vi "GoTo.vi"(7 "theta":dbl, 8 "error in (no error)":errorcluster, 9 "Position":cluster{"X":dbl, "Y":dbl, "Theta":dbl}, 10 "y path":i32[](array[numeric]), 11 "x path":i32[](array[numeric])) -> (0 "Error/Flow Out":errorcluster, 1 "New Position":cluster{"X":dbl, "Y":dbl, "Theta":dbl})   [LabVIEW 2018]
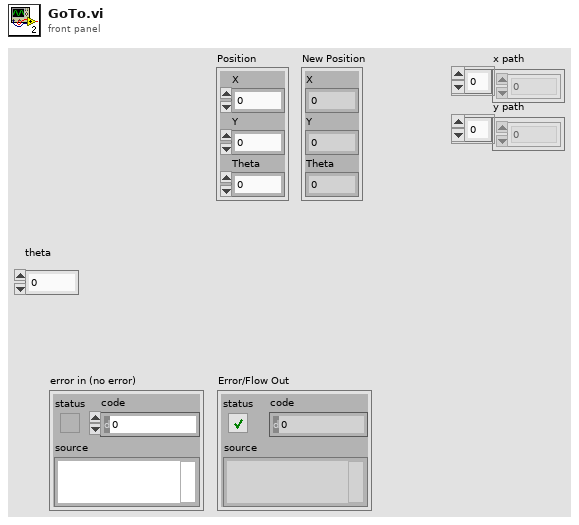
[diagram p1: front panel]
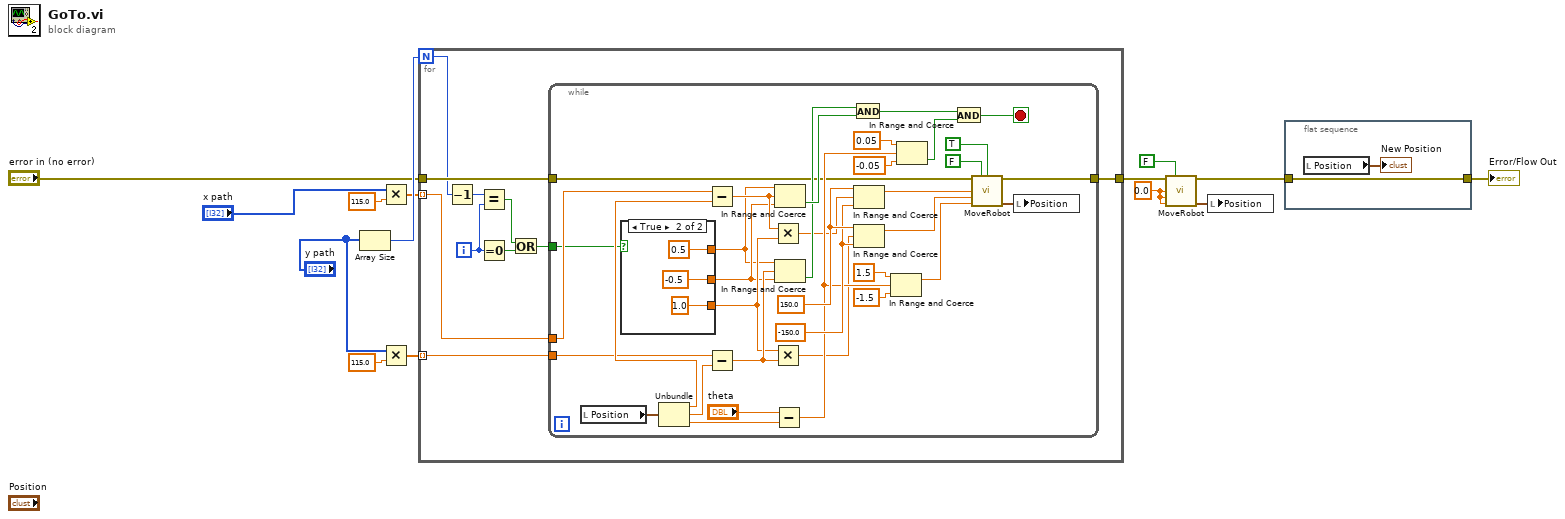
[diagram p0: block diagram]
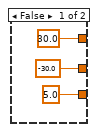
[diagram p2: hidden frame]
diagram:
  w6 = 0.0 ("x (mm/s)")
  n1 = Array Size(array="y path") -> (size(s)=w10:i32)
  n2 = Multiply(x="x path", y=115.0) -> (x*y=w8:dbl[])
  n3 = Multiply(x="y path", y=115.0) -> (x*y=w9:dbl[])
  n4 = for {
    N: w10 -> [w20]
    tunnel: w9 -> [w23] mode=indexing
    tunnel: w8 -> [w24] mode=indexing
    tunnel: "error in (no error)" -> [w22]
    tunnel: [w21] -> w5
    i -> [w18]
    n5 = Decrement(x=w20) -> (x-1=w19:i32)
    n6 = Equal?(x=w19, y=w18) -> (x = y?=w16:bool)
    n7 = Equal To 0?(x=w18) -> (x = 0?=w17:bool)
    n8 = Or(x=w16, y=w17) -> (x .or. y?=w15:bool)
    n9 = while {
      tunnel: w24 -> [w58]
      tunnel: w23 -> [w56]
      tunnel: w22 -> [w38]
      tunnel: [w35] -> w21
      tunnel: w15 -> [w25]
      stop <- w49 stop-if-true
      w43 = -150.0 ("lower limit")
      w44 = 150.0 ("upper limit")
      n10 = local read "Position"() -> (w59:cluster{"X":dbl, "Y":dbl, "Theta":dbl})
      n11 = case shown="True" w25 {
        tunnel: [5.0 ("y") 1.0 ("y")] -> w28
        tunnel: [-30.0 ("lower limit") -0.5 ("lower limit")] -> w27
        tunnel: [30.0 ("upper limit") 0.5 ("upper limit")] -> w26
        frame False {
        }
        frame True {
        }
      }
      n12 = Unbundle(w59) -> ("X"=w57:dbl, "Y"=w55:dbl, "Theta"=w53:dbl)
      n13 = Subtract(x=w58, y=w57) -> (x-y=w31:dbl)
      n14 = Subtract(x=w56, y=w55) -> (x-y=w29:dbl)
      n15 = Multiply(x=w31, y=w28) -> (x*y=w32:dbl)
      n16 = Multiply(x=w28, y=w29) -> (x*y=w30:dbl)
      n17 = Subtract(x="theta", y=w53) -> (x-y=w40:dbl)
      n18 = In Range and Coerce(upper limit=w26, x=w31, lower limit=w27) -> (In Range?=w52:bool)  [unwired: 1 out]
      n19 = In Range and Coerce(upper limit=w26, x=w29, lower limit=w27) -> (In Range?=w51:bool)  [unwired: 1 out]
      n20 = And(x=w51, y=w52) -> (x .and. y?=w50:bool)
      n21 = In Range and Coerce(upper limit=w44, x=w32, lower limit=w43) -> (coerced(x)=w46:dbl)  [unwired: 1 out]
      n22 = In Range and Coerce(upper limit=w44, x=w30, lower limit=w43) -> (coerced(x)=w45:dbl)  [unwired: 1 out]
      n23 = In Range and Coerce(upper limit=1.5, x=w40, lower limit=-1.5) -> (coerced(x)=w39:dbl)  [unwired: 1 out]
      n24 = In Range and Coerce(upper limit=0.05, x=w40, lower limit=-0.05) -> (In Range?=w34:bool)  [unwired: 1 out]
      n25 = And(x=w50, y=w34) -> (x .and. y?=w49:bool)
      n26 = call "MoveRobot.vi"("Error/Flow In"=w38, "Reset"=FALSE, "Relative to Global Frame"=TRUE, "x (mm/s)"=w46, "y (mm/s)"=w45, "theta (rad/s)"=w39) -> ("Error/Flow Out"=w35:errorcluster, "Position"=w33:cluster{"X":dbl, "Y":dbl, "Theta":dbl})  [unwired: 8 in]
      n27 = local write "Position"(w33) -> ()
    }
  }
  n28 = call "MoveRobot.vi"("Error/Flow In"=w5, "Reset"=FALSE, "x (mm/s)"=w6, "y (mm/s)"=w6, "theta (rad/s)"=w6) -> ("Error/Flow Out"=w3:errorcluster, "Position"=w4:cluster{"X":dbl, "Y":dbl, "Theta":dbl})  [unwired: 9 in]
  n29 = local write "Position"(w4) -> ()
  n30 = flat-sequence {
    tunnel: w3 -> [w66]
    tunnel: [w66] -> w2
    frame #0 {
      n31 = local read "Position"() -> (→"New Position":cluster{"X":dbl, "Y":dbl, "Theta":dbl})
    }
  }
  "Error/Flow Out" <- w2
